vi "Write Dynamic RPTID File.vi"(8 "error in (no error)":errorcluster, 11 "RPTID Data In":T1[](array[typedef])) -> (0 "error out":errorcluster)   [LabVIEW 2020, in "SECS Communication.lvlib" / "SECS Data Class.lvclass"]
uses:
  SECS Data Class.lvclass
  RPTID Data.ctl
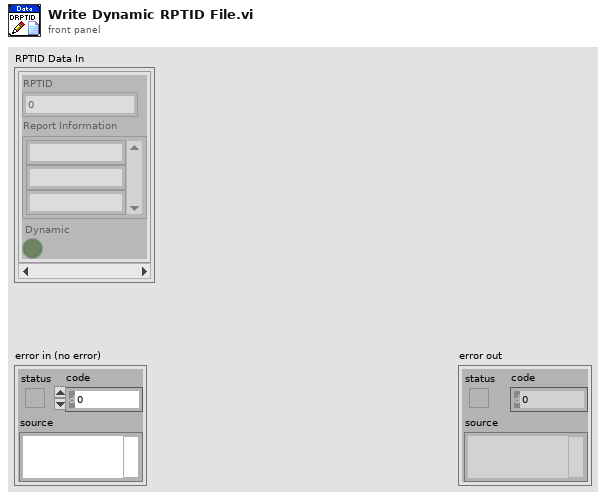
[diagram p1: front panel]
types:
  T1 = typedef "SECS Communication.lvlib/SECS Data Class.lvclass/RPTID Data.ctl" = cluster{"RPTID":u32, "Report Information":string[], "Dynamic":bool}
  T2 = enum16{"open", "replace", "create", "open or create", "replace or create", "replace or create with confirmation"}
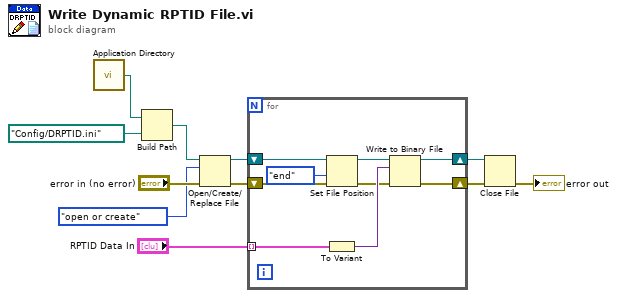
[diagram p0: block diagram]
diagram:
  n1 = call <vilib>:"Application Directory.vi"() -> ("Application Directory"=w11:path)
  n2 = Build Path(base path=w11, name or relative path=path "Config/DRPTID.ini") -> (appended path=w8:path)
  n3 = Open/Create/Replace File(file path (use dialog)=w8, error in="error in (no error)", operation (0:open)=T2."open or create") -> (refnum out=w5:refnum<file>, error out=w4:errorcluster)  [unwired: 3 in, 1 out]
  n4 = for {
    tunnel: "RPTID Data In" -> [w20] mode=indexing
    shift-right: [w18] -> w3
    shift-left: w5 -> [w16]
    shift-right: [w12] -> w2
    shift-left: w4 -> [w15]
    n5 = Set File Position(refnum=w16, from (0:start)=enum16{"start", "end", "current"}."end", error in=w15) -> (refnum out=w13:refnum<file>, error out=w14:errorcluster)  [unwired: 1 in]
    n6 = To Variant(anything=w20) -> (Variant=w19:variant)
    n7 = Write to Binary File(file (use dialog)=w13, data=w19, error in=w14) -> (refnum out=w18:refnum<file>, error out=w12:errorcluster)  [unwired: 3 in, 1 out]
  }
  n8 = Close File(refnum=w3, error in=w2) -> (error out=→"error out":errorcluster)  [unwired: 1 out]
